vi "Error if Invalid.vi"(8 "error in (no error)":errorcluster, 11 "SQLite3LV Cursor in":refnum<class "cursor.lvclass">) -> (0 "error out":errorcluster, 3 "SQLite3LV Cursor out":refnum<class "cursor.lvclass">)   [LabVIEW 2014, in "SQLite3LV.lvlib" / "cursor.lvclass"]
uses:
  cursor.lvclass
  cursor.lvclass/cursor.ctl
  SQLite3 Class/sqlite3.lvclass/sqlite3.ctl
  SQLite3 Class/sqlite3.lvclass
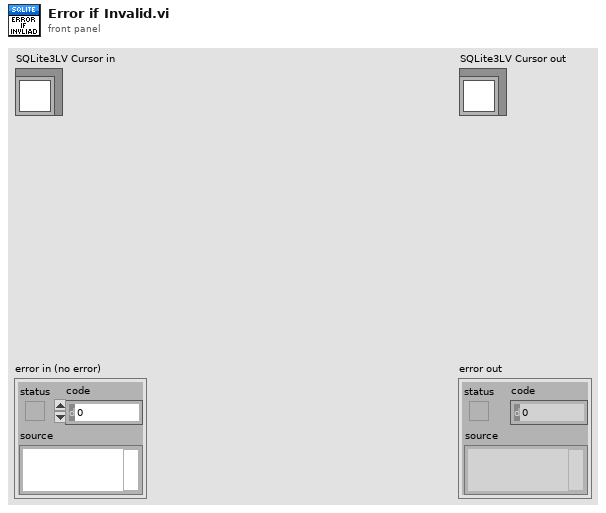
[diagram p1: front panel]
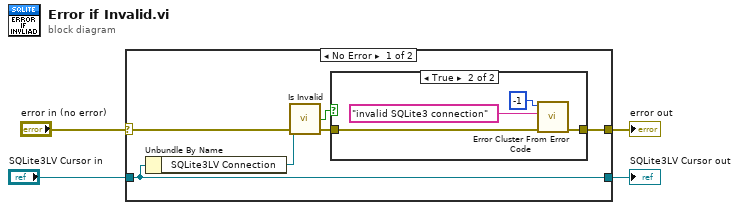
[diagram p0: block diagram]
diagram:
  n1 = case shown="No Error" "error in (no error)" {
    selector: "error in (no error)" -> [w7 w17]
    tunnel: [w5 w17] -> w3
    tunnel: [w10 w16] -> w1
    tunnel: "SQLite3LV Cursor in" -> [w10 w16]
    frame No Error {
      n2 = Unbundle By Name(w10) -> ("SQLite3LV Connection"=w9:refnum<class "sqlite3.lvclass">)
      n3 = call "Is Invalid.vi"("error in (no error)"=w7, "SQLite3LV Connection in"=w9) -> ("error out"=w6:errorcluster, "not a database"=w8:bool)  [unwired: 2 in]
      n4 = case shown="True" w8 {
        tunnel: w6 -> [w11 w13]
        tunnel: [w11 w12] -> w5
        frame False {
        }
        frame True {
          n5 = call <vilib>:"Error Cluster From Error Code.vi"("error in (no error)"=w13, "error message (\"\")"="invalid SQLite3 connection" ("error message (\"\")"), "error code (0)"=-1) -> ("error out"=w12:errorcluster)  [unwired: 6 in]
        }
      }
    }
    frame Error {
    }
  }
  "error out" <- w3
  "SQLite3LV Cursor out" <- w1
